vi "Filter Material Type String.vi"(8 "error in (no error)":errorcluster, 10 "Material Type":string, 11 "Application in":refnum<class "Application.lvclass">) -> (0 "error out":errorcluster, 2 "Filtered Material Type":string, 3 "Application out":refnum<class "Application.lvclass">)   [LabVIEW 2017, in "Application.lvlib" / "Application.lvclass"]
doc: "Removes common add-on characters from a Material Type string identifier. If they're not present string is left unchagned."
uses:
  Application.lvclass
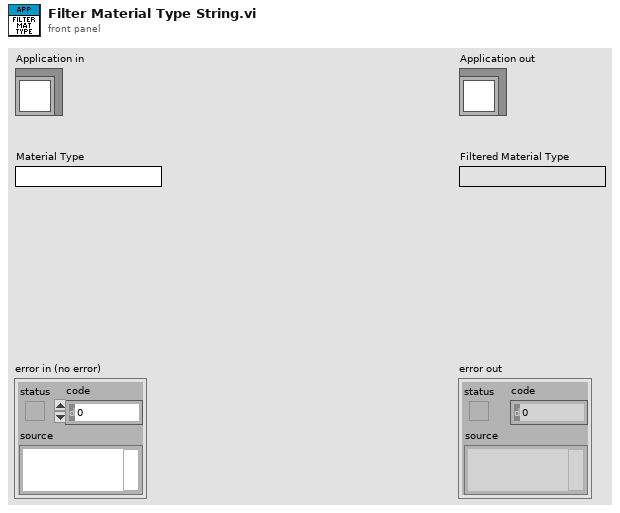
[diagram p1: front panel]
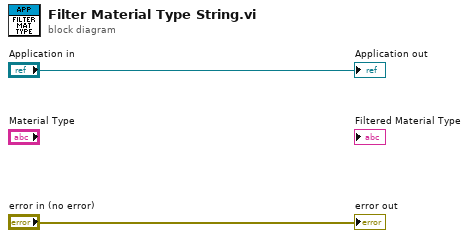
[diagram p0: block diagram]
diagram:
  "error out" <- "error in (no error)"
  "Application out" <- "Application in"
